vi "Close Connection.vi"(8 "Error In":errorcluster, 11 "SqlMapper":refnum<class "SqlMapper.lvclass">) -> (0 "Error Out":errorcluster)   [LabVIEW 2020, in "ORM_API.lvlib"]
uses:
  ORM_API.lvlib
  <vilib>/Viviota/shared/ORM.lvlibp/ORM/SqlMapper/SqlMapper.lvclass
  <vilib>/Viviota/shared/ORM.lvlibp/ORM/SqlMapper/Read DbConnection.vi
  <vilib>/Viviota/shared/ORM.lvlibp/ORM/DbConnection/DbConnection.lvclass
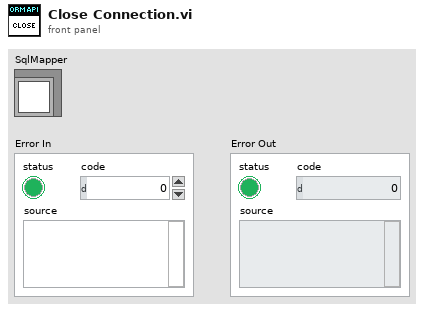
[diagram p1: front panel]
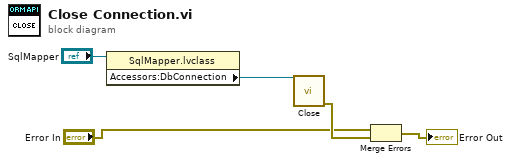
[diagram p0: block diagram]
diagram:
  n1 = property class="SqlMapper.lvclass"(reference="SqlMapper") -> ("Accessors:DbConnection"=w4:refnum<class "DbConnection.lvclass">)  [unwired: 1 in, 2 out]
  n2 = call-dynamic "Close.vi"("DbConnection in"=w4) -> ("error out"=w3:errorcluster)  [unwired: 10 in]
  n3 = Merge Errors("Error In", w3) -> (→"Error Out":errorcluster)
